vi "Set_Wave_Keithley6221.vi"(9 "Error in":errorcluster) -> (3 "Erro out":errorcluster)   [LabVIEW 2016]
uses:
  Equipment/Keithley 622x/Configure/6221 Wave/Low Level/Typedefs/KE6221 -- Wave Type tmp.ctl
  Instrument_Setup.vi
  Global/Global Variables/Data_Display_global.vi
  Equipment/Keithley 622x/Keithley 622x tmp.lvlib
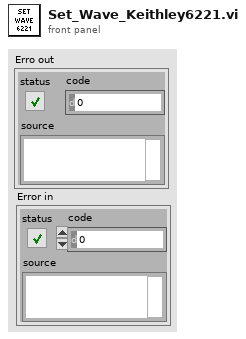
[diagram p1: front panel]
types:
  T1 = typedef "Keithley 622x tmp.lvlib/KE6221 -- Wave Type tmp.ctl" = enum16{"Sinusoid", "Square", "Ramp", "Arbitrary 0", "Arbitrary 1", "Arbitrary 2", "Arbitrary 3", "Arbitrary 4"}
  T2 = typedef "Keithley 622x tmp.lvlib/KE6221 -- Wave Sine Wave Params tmp.ctl" = cluster{"Frequency (Hz)":T3, "Amplitude (A)":T4, "Offset (A)":T5, "Ranging Mode":T6, "Fixed Range":T7, "Playback Mode":T8, "Time (s)":T9, "Num Cycles":T10, "Phase\nMarker?":bool, "Phase Marker (deg)":T11, "Trig Link Line":T12}
  T3 = typedef "Keithley 622x tmp.lvlib/KE6221 -- Wave Frequency tmp.ctl" = dbl
  T4 = typedef "Keithley 622x tmp.lvlib/KE6221 -- Wave Amplitude tmp.ctl" = dbl
  T5 = typedef "Keithley 622x tmp.lvlib/KE622x -- Current Level tmp.ctl" = dbl
  T6 = typedef "Keithley 622x tmp.lvlib/KE6221 -- Wave Ranging Mode tmp.ctl" = enum16{"Best", "Fixed"}
  T7 = typedef "Keithley 622x tmp.lvlib/KE622x -- Current Ranges tmp.ctl" = enum16{"2nA", "20nA", "200nA", "2uA", "20uA", "200uA", "2mA", "20mA", "100mA"}
  T8 = typedef "Keithley 622x tmp.lvlib/KE6221 -- Wave Playback Mode tmp.ctl" = enum16{"Time", "Num Cycles"}
  T9 = typedef "Keithley 622x tmp.lvlib/KE6221 -- Wave Playback Time tmp.ctl" = dbl
  T10 = typedef "Keithley 622x tmp.lvlib/KE6221 -- Wave Playback Num Cycles tmp.ctl" = dbl
  T11 = typedef "Keithley 622x tmp.lvlib/KE6221 -- Wave Phase Marker tmp.ctl" = dbl
  T12 = typedef "Keithley 622x tmp.lvlib/KE622x -- Trig Link Line tmp.ctl" = enum16{"1", "2", "3", "4", "5", "6"}
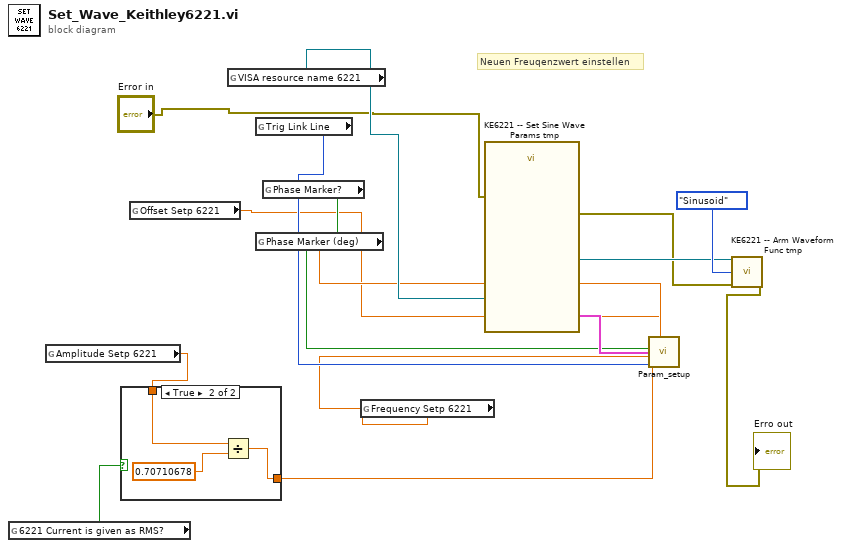
[diagram p0: block diagram]
diagram:
  # "Neuen Freuqenzwert einstellen"
  n1 = global read "Instrument_Setup.vi" "6221 Current is given as RMS?"() -> (w2:bool)
  n2 = global read "Data_Display_global.vi" "Amplitude Setp 6221"() -> (w4:dbl)
  n3 = case shown="True" w2 {
    tunnel: [w16 w19] -> w3
    tunnel: w4 -> [w16 w18]
    frame False {
    }
    frame True {
      n4 = Divide(x=w18, y=0.70710678) -> (x/y=w19:dbl)
    }
  }
  n5 = global read "Data_Display_global.vi" "Offset Setp 6221"() -> (w1:dbl)
  n6 = global read "Instrument_Setup.vi" "VISA resource name 6221"() -> (w15:refnum<visa-resource-name>)
  n7 = global read "Instrument_Setup.vi" "Trig Link Line"() -> (w12:i32)
  n8 = global read "Instrument_Setup.vi" "Phase Marker (deg)"() -> (w11:dbl)
  n9 = global read "Instrument_Setup.vi" "Phase Marker?"() -> (w13:bool)
  n10 = global read "Data_Display_global.vi" "Frequency Setp 6221"() -> (w7:dbl)
  n11 = call "Param_setup.vi"("Offset"=w1, "Phase Marker (deg)"=w11, "Trig Link Line"=w12, "Frequency"=w7, "Phase Marker?"=w13, "Amplitude"=w3) -> ("Sine Wave Params 2"=w14:T2)
  n12 = call "KE6221 -- Set Sine Wave Params tmp.vi"("Resource In"=w15, "Sine Wave Params In"=w14, "error in (no error)"="Error in") -> ("Resource Out (dupl)"=w9:refnum<visa-resource-name>, "error out"=w8:errorcluster)  [unwired: 10 in, 1 out]
  n13 = call "KE6221 -- Arm Waveform Func tmp.vi"("Resource In"=w9, "Wave Type"=KE6221_--_Wave_Type_tmp."Sinusoid", "error in (no error)"=w8) -> ("error out"=→"Erro out":errorcluster)  [unwired: 11 in, 1 out]
